vi "VMI_acquire_rewrite.vi"(0 "IO settings":T1, 1 "Queue Array":T7[](array[typedef]), 3 "Peak Find Settings":T5, 9 "Collection Information":T6[](array[typedef]), 11 "error in":errorcluster, 12 "Collect_refs":T4, 14 "Big_image Array":i16[][][](array[numeric])) -> (4 "Histogram":i32[][](array[numeric]), 6 "Peak Array":cluster{"X":sgl, "Y":sgl}[][](array[cluster]), 8 "Powers":dbl[][](array[numeric]), 10 "Power Err":dbl[][](array[numeric]), 15 "error IO":errorcluster)   [LabVIEW 2015]
doc: "This VI collects the images, finds the number of counts in each image"
uses:
  Type defs/FileAcq_v1_Ctrl.ctl
  Type defs/VMI_collection_refs.ctl
  Type defs/IO_settings_ctrl.ctl
  <vilib>/vision/Image Controls.llb/IMAQ Image.ctl
  <vilib>/userdefined/High Color/IMAQdx.ctl
panel:
  out "xaxis":i32[][](array[numeric])
  out "XY Graph":cluster{"Y":dbl[], "Y":dbl[]}[](graph)
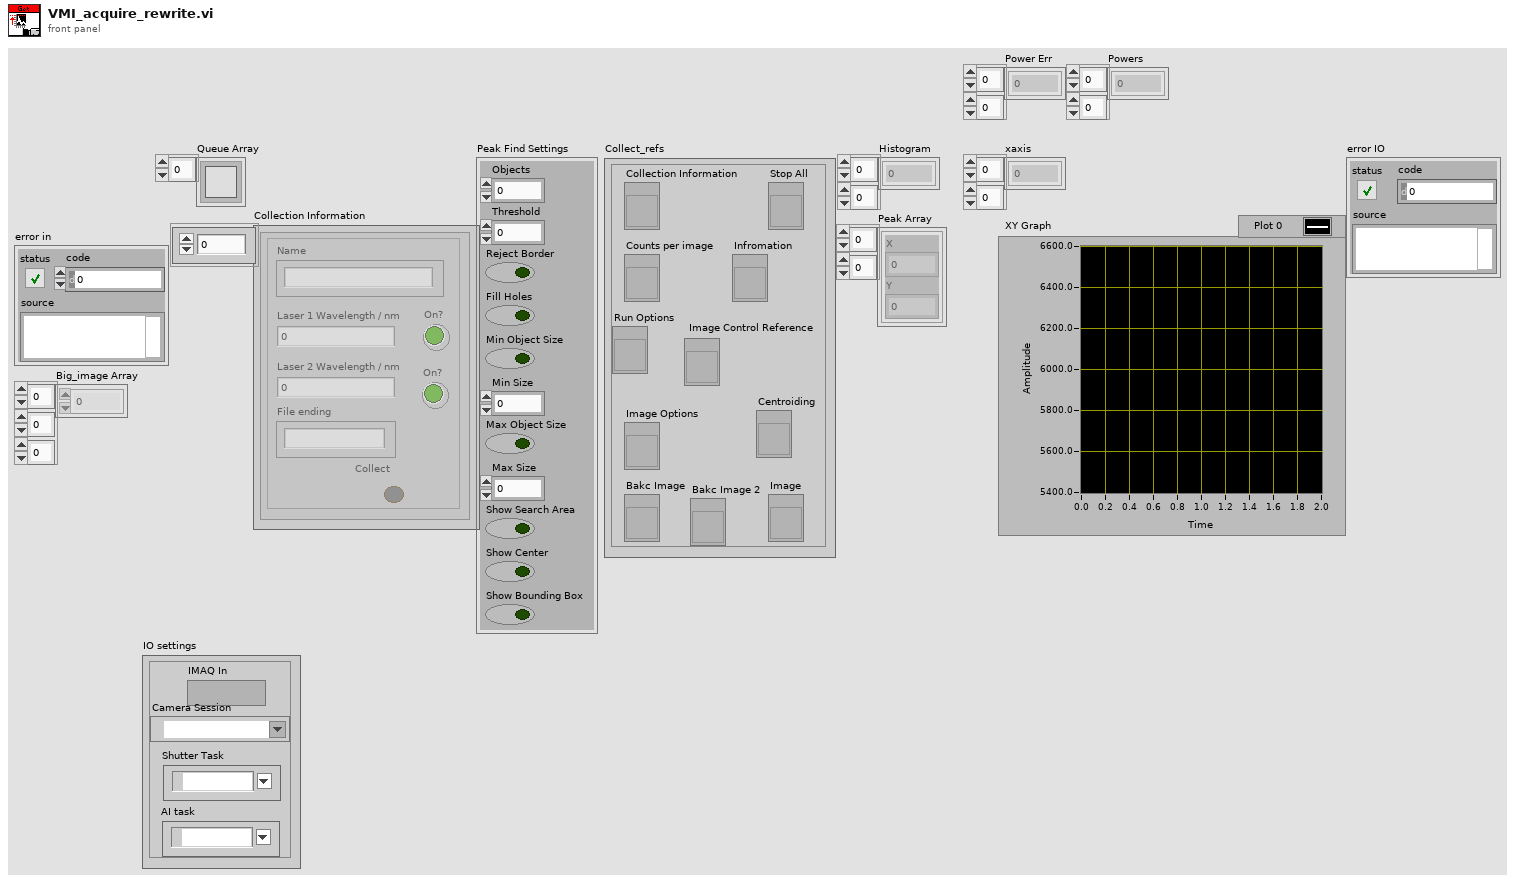
[diagram p1: front panel]
types:
  T1 = typedef "IO_settings_ctrl.ctl" = cluster{"IMAQ In":T2, "Camera Session":T3, "Shutter Task":refnum<k21>, "AI task":refnum<k21>}
  T2 = typedef "IMAQ Image.ctl" = refnum<image>
  T3 = typedef "IMAQdx.ctl" = refnum<k21>
  T4 = typedef "VMI_collection_refs.ctl" = cluster{"Stop All":refnum<vi>, "Collection Information ":refnum<vi>, "Infromation":refnum<vi>, "Counts per image":refnum<vi>, " Image Control Reference ":refnum<vi>, "Run Options":refnum<vi>, "Image Options":refnum<vi>, "Centroiding":refnum<vi>, "Image":refnum<vi>, "Bakc Image":refnum<vi>, "Bakc Image 2":refnum<vi>}
  T5 = cluster{"Objects":u16, "Threshold":i32, "Reject Border":bool, "Fill Holes":bool, "Min Object Size":bool, "Min Size":i32, "Max Object Size":bool, "Max Size":i32, "Show Search Area":bool, "Show Center":bool, "Show Bounding Box":bool}
  T6 = typedef "FileAcq_v1_Ctrl.ctl" = cluster{"Type":string, "LaserWave1":dbl, "Shutter1":bool, "LaserWave2":dbl, "Shutter2":bool, "FileEnd":string, "Collect":bool}
  T7 = typedef "Queue RefNum" = refnum<k1>
  T8 = typedef "Image Type" = u32
  T9 = cluster{"Total Time / ms":dbl, "Image Total Collection Time":dbl, "Image Loop time / ms":dbl, "Peak Total Find Time":dbl, "Peak Find Time / ms":dbl, "Camera Rate / Hz":dbl, "Total Number of Loops":dbl, "Current Loop Number":dbl, "Number of Image Loops":dbl, "Run Mode":dbl}
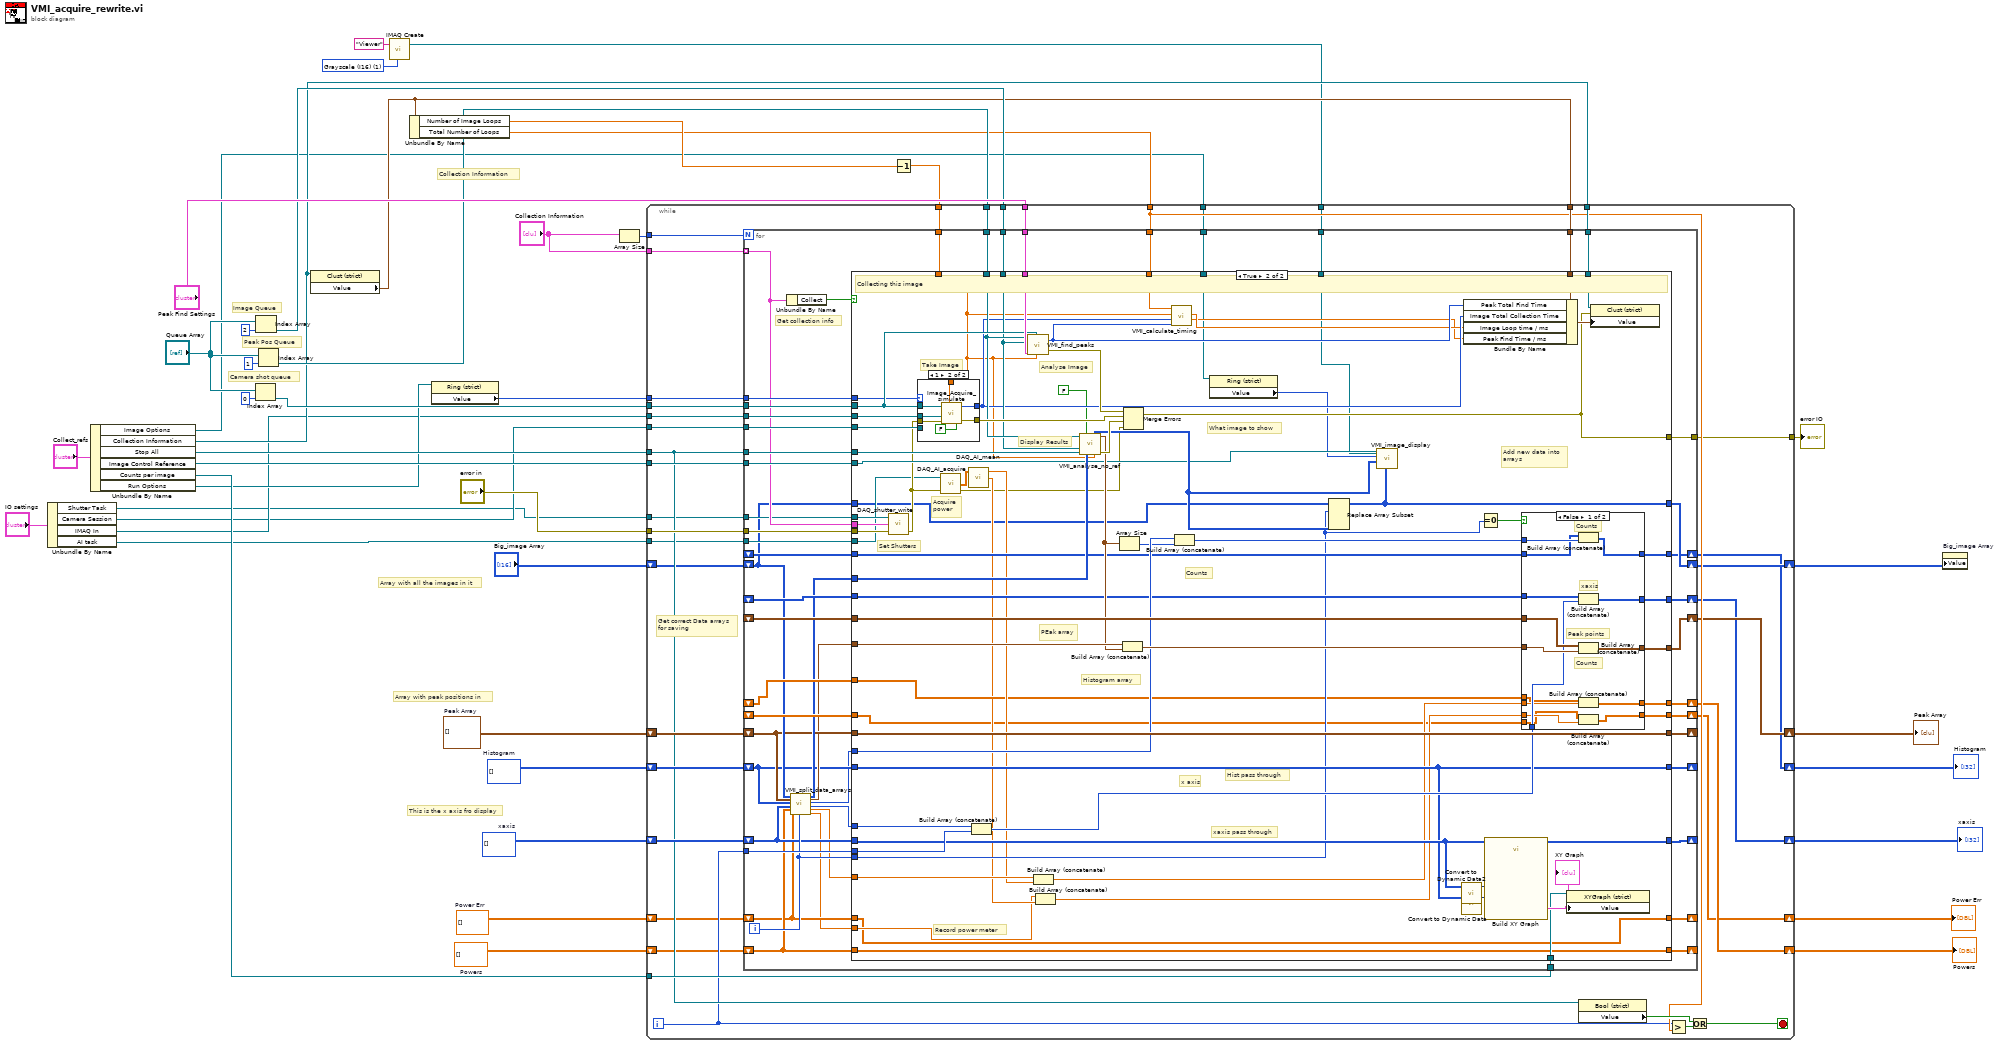
[diagram p0: block diagram]
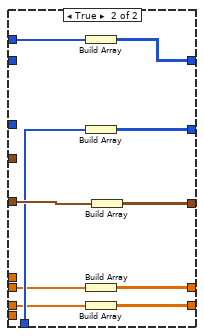
[diagram p3: hidden frame]
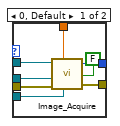
[diagram p4: hidden frame]
diagram:
  w3 = dbl[][] []  # Power Err
  w4 = dbl[][] []  # Powers
  w13 = T8 1 items=["Grayscale (U8)", "Grayscale (I16)", "Grayscale (SGL)", "Complex (CSG)", "RGB (U32)", "HSL (U32)", "RGB (U64)", "Grayscale (U16)"] ("Image Type")
  w5 = i32[][] []  # xaxis
  w23 = i32[][] []  # Histogram
  w25 = cluster{"X":sgl, "Y":sgl}[][] []  # Peak Array
  # "Array with all the images in it"
  # "Array with peak positions in"
  # "This is the x axis fro display"
  # "Collection Information"
  # "Image Queue"
  # "Peak Pos Queue"
  # "Camera shot queue"
  n1 = Unbundle By Name("IO settings") -> ("Shutter Task"=w7:refnum<k21>, "Camera Session"=w8:T3, "IMAQ In"=w9:T2, "AI task"=w6:refnum<k21>)
  n2 = Unbundle By Name("Collect_refs") -> ("Image Options"=w11:refnum<vi>, "Collection Information"=w27:refnum<vi>, "Stop All"=w33:refnum<vi>, "Image Control Reference"=w32:refnum<vi>, "Counts per image"=w24:refnum<vi>, "Run Options"=w16:refnum<vi>)
  n3 = Index Array(array="Queue Array", index=0) -> (element=w42:T7)
  n4 = Index Array(array="Queue Array", index=2) -> (element=w35:T7)
  n5 = Index Array(array="Queue Array", index=1) -> (element=w38:T7)
  n6 = property class="Clust (strict)"(reference=w27) -> ("Value"=w28:T9)  [unwired: 1 in, 2 out]
  n7 = call "IMAQ Create"("Image Name"="Viewer", "Image Type"=w13) -> ("New Image"=w12:T2)  [unwired: 3 in, 1 out]
  n8 = Unbundle By Name(w28) -> ("Number of Image Loops"=w31:dbl, "Total Number of Loops"=w29:dbl)
  n9 = property class="Ring (strict)"(reference=w16) -> ("Value"=w15:u16)  [unwired: 1 in, 2 out]
  n10 = Array Size(array="Collection Information") -> (size(s)=w26:i32)
  n11 = Decrement(x=w31) -> (x-1=w30:dbl)
  n12 = while {
    tunnel: w9 -> [w82]
    tunnel: w8 -> [w81]
    tunnel: "error in" -> [w80]
    tunnel: w42 -> [w79]
    tunnel: "Collection Information" -> [w78]
    tunnel: "Peak Find Settings" -> [w77]
    tunnel: w38 -> [w76]
    tunnel: w35 -> [w75]
    tunnel: w33 -> [w66]
    tunnel: w32 -> [w74]
    tunnel: w30 -> [w73]
    tunnel: w29 -> [w63]
    tunnel: w28 -> [w72]
    tunnel: w27 -> [w71]
    tunnel: w26 -> [w56]
    tunnel: w24 -> [w68]
    shift-right: [w55] -> w17
    shift-left: w25 -> [w70]
    shift-right: [w54] -> w18
    shift-left: w23 -> [w67]
    shift-right: [w53] -> w22
    shift-left: w5 -> [w69]
    tunnel: [w62] -> w21
    shift-right: [w61] -> w19
    shift-left: "Big_image Array" -> [w59]
    tunnel: w15 -> [w58]
    tunnel: w12 -> [w52]
    tunnel: w11 -> [w51]
    tunnel: w7 -> [w50]
    tunnel: w6 -> [w49]
    shift-right: [w46] -> w1
    shift-left: w4 -> [w48]
    shift-right: [w45] -> w2
    shift-left: w3 -> [w47]
    i -> [w60]
    stop <- w57 stop-if-true
    # "Get correct Data arrays\nfor saving"
    n13 = for {
      N: w56 -> [_]
      tunnel: w82 -> [w134]
      tunnel: w81 -> [w133]
      tunnel: w80 -> [w132]
      tunnel: w79 -> [w131]
      tunnel: w78 -> [w104] mode=indexing
      tunnel: w77 -> [w129]
      tunnel: w76 -> [w128]
      tunnel: w75 -> [w127]
      tunnel: w66 -> [w126]
      tunnel: w74 -> [w125]
      tunnel: w73 -> [w123]
      tunnel: w63 -> [w122]
      tunnel: w60 -> [w119]
      tunnel: w72 -> [w121]
      tunnel: w71 -> [w120]
      tunnel: w68 -> [w118]
      shift-right: [w117] -> _
      shift-left: w70 -> [w92]
      shift-right: [w124] -> _
      shift-left: w67 -> [w90]
      shift-right: [w116] -> _
      shift-left: w69 -> [w88]
      tunnel: [w115] -> w62
      shift-right: [w114] -> w61
      shift-left: w59 -> [w94]
      tunnel: w58 -> [w113]
      shift-right: [w112] -> w55
      shift-left: _ -> [w111]
      shift-right: [w110] -> w54
      shift-left: _ -> [w109]
      shift-right: [w108] -> w53
      shift-left: _ -> [w107]
      tunnel: w52 -> [w106]
      tunnel: w51 -> [w105]
      tunnel: w50 -> [w103]
      tunnel: w49 -> [w102]
      shift-right: [w101] -> _
      shift-left: w48 -> [w86]
      shift-right: [w100] -> w46
      shift-left: _ -> [w99]
      shift-right: [w98] -> _
      shift-left: w47 -> [w85]
      shift-right: [w97] -> w45
      shift-left: _ -> [w96]
      i -> [w95]
      # "Get collection info"
      # "This loop collects for each required image"
      n14 = Unbundle By Name(w104) -> ("Collect"=w130:bool)
      n15 = call "VMI_split_data_arrays.vi"("Big_image Array in"=w94, "Peak Array in"=w92, "Histogram in"=w90, "xaxis in"=w88, "Powers in"=w86, "Power Err in"=w85, "ArrayIndex"=w95) -> ("Big_image Array out"=w93:i16[][], "Peak Array out"=w91:cluster{"X":sgl, "Y":sgl}[], "Histogram out"=w89:i32[], "xaxis out"=w87:i32[], "Powers out"=w84:dbl[], "Power Err out"=w83:dbl[])  [unwired: 7 in]
      n16 = case shown="True" w130 {
        tunnel: w134 -> [_ w216]
        tunnel: w133 -> [_ w215]
        tunnel: w132 -> [w143 w163]
        tunnel: w131 -> [_ w213]
        tunnel: w129 -> [_ w214]
        tunnel: w128 -> [_ w210]
        tunnel: w127 -> [_ w209]
        tunnel: w126 -> [_ w208]
        tunnel: w125 -> [_ w168]
        tunnel: [w143 w196] -> w115
        tunnel: w91 -> [_ w185]
        tunnel: w92 -> [w141 w186]
        tunnel: [w141 w186] -> w117
        tunnel: w90 -> [w140 w171]
        tunnel: w89 -> [_ w182]
        tunnel: [w140 w171] -> w124
        tunnel: w123 -> [_ w190]
        tunnel: w122 -> [_ w207]
        tunnel: w119 -> [_ w173]
        tunnel: w87 -> [_ w175]
        tunnel: w88 -> [w139 w172]
        tunnel: [w139 w172] -> w116
        tunnel: w121 -> [_ w203]
        tunnel: w120 -> [_ w197]
        tunnel: w95 -> [_ w169]
        tunnel: w118 -> [_ w194]
        tunnel: w94 -> [w142 w145]
        tunnel: [w142 w144] -> w114
        tunnel: w93 -> [_ w193]
        tunnel: w113 -> [_ w192]
        tunnel: [w141 w188] -> w112
        tunnel: w111 -> [_ w187]
        tunnel: [w140 w179] -> w110
        tunnel: w109 -> [_ w178]
        tunnel: [w139 w177] -> w108
        tunnel: w107 -> [_ w176]
        tunnel: w106 -> [_ w167]
        tunnel: w105 -> [_ w166]
        tunnel: w104 -> [_ w164]
        tunnel: w103 -> [_ w162]
        tunnel: w102 -> [_ w160]
        tunnel: w84 -> [_ w157]
        tunnel: w86 -> [w138 w158]
        tunnel: [w138 w158] -> w101
        tunnel: [w136 w155] -> w100
        tunnel: w99 -> [w136 w154]
        tunnel: w83 -> [_ w151]
        tunnel: w85 -> [w137 w150]
        tunnel: [w137 w150] -> w98
        tunnel: [w135 w148] -> w97
        tunnel: w96 -> [w135 w147]
        frame False {
          # "Not collecting this image"
        }
        frame True {
          # "xaxis pass through"
          # "Hist pass through"
          # "Acquire\npower"
          # "Record power meter"
          # "Set Shutters"
          # "What image to show"
          # "x axis"
          # "Histogram array"
          # "PEak array"
          # "Counts"
          # "Add new data into\narrays"
          # "Display Results"
          # "Analyse Image"
          # "Take Image"
          # "Collecting this image"
          n17 = call "DAQ_shutter_write.vi"("Error In"=w163, "Collection Settings"=w164, "DAQmx Task Name"=w162) -> ("Error Out"=w161:errorcluster)  [unwired: 2 in]
          n18 = case shown="1" w192 {
            tunnel: w216 -> [w248 w250]
            tunnel: w215 -> [w247 _]
            tunnel: w161 -> [w246 w256]
            tunnel: w213 -> [w245 w252]
            tunnel: [w244 w255] -> w211
            tunnel: w190 -> [w243 w253]
            tunnel: [w242 w254] -> w201
            frame 0, Default {
              n19 = call "Image_Acquire.vi"("Queue Ref in"=w245, "Acquire Time"=w243, "Image Out"=w248, "Session In"=w247, "error in (no error)"=w246, "Test Timing"=FALSE) -> ("Loop Time Out"=w242:i64, "error out"=w244:errorcluster)  [unwired: 1 in]
            }
            frame 1 {
              n20 = call "Image_Acquire_simulate.vi"("Queue Ref in"=w252, "Acquire Time"=w253, "Image Out"=w250, "error in (no error)"=w256, "Test Timing"=FALSE) -> ("Loop Time Out"=w254:i64, "error out"=w255:errorcluster)  [unwired: 2 in]
            }
          }
          n21 = call "DAQ_AI_acquire.vi"("Error In"=w161, "DAQmx Task Name"=w160) -> ("Error Out"=w146:errorcluster, "data"=w159:dbl[][])  [unwired: 1 in, 1 out]
          n22 = call "DAQ_AI_mean.vi"("data"=w159) -> ("Std"=w152:dbl[], "Mean"=w156:dbl[])  [unwired: 3 in]
          n23 = Build Array (concatenate)(w175, w173) -> (w174:i32[])
          n24 = call "VMI_find_peaks.vi"("Acquire Time"=w190, "Acquire Queue In"=w213, "Peak Find Settings"=w214, "Image Queue in"=w209, "Peak Position Queue in"=w210) -> ("error out"=w212:errorcluster, "x-y"=w202:u32)  [unwired: 1 in]
          n25 = Build Array (concatenate)(w157, w156) -> (w153:dbl[])
          n26 = Build Array (concatenate)(w151, w152) -> (w149:dbl[])
          n27 = call "VMI_analyse_no_ref.vi"("Peak Position Queue in"=w210, "Test Timing"=FALSE, "Image in"=w209, "Stop Button Ref"=w208, "Image_array"=w193, "Acquire Time"=w190) -> ("Image_array out"=w170:i32[][], "Peaks Position Out"=w184:cluster{"X":sgl, "Y":sgl}[], "error out"=w205:errorcluster)  [unwired: 5 in, 2 out]
          n28 = Array Size(array=w184) -> (size(s)=w181:i32)
          n29 = Build Array (concatenate)(w185, w184) -> (w183:cluster{"X":sgl, "Y":sgl}[])
          n30 = Merge Errors(w212, w211, w205, w146) -> (w196:errorcluster)
          n31 = call "VMI_calculate_timing.vi"("Peakfind total time"=w202, "Camera_Total_loop time"=w201, "Number of image loops"=w190, "Total loop Number"=w207) -> ("AveragePeak find time"=w199:dbl, "Average Image Loop time"=w200:dbl)  [unwired: 1 in, 1 out]
          n32 = Build Array (concatenate)(w182, w181) -> (w180:i32[])
          n33 = property class="Ring (strict)"(reference=w166) -> ("Value"=w165:u16)  [unwired: 1 in, 2 out]
          n34 = Replace Array Subset(array=w145, new element=w170, index (dim 0)=w169) -> (w144:i16[][][])  [unwired: 2 in]
          n35 = call "VMI_image_display.vi"("Image_control"=w168, "Image to show"=w165, "Current Image"=w170, "Big_image Array"=w144, "Canvas"=w167) -> ()  [unwired: 5 in, 1 out]
          n36 = call "Convert to Dynamic Data2"("2D Array"=w172) -> ("Dynamic Data Type"=w204:dynamicdata)  [unwired: 3 in]
          n37 = call "Convert to Dynamic Data"("2D Array"=w171) -> ("Dynamic Data Type"=w206:dynamicdata)  [unwired: 3 in]
          n38 = Bundle By Name(cluster=w203, "Peak Total Find Time"=w202, "Image Total Collection Time"=w201, "Image Loop time / ms"=w200, "Peak Find Time / ms"=w199) -> (w198:T9)
          n39 = Equal To 0?(x=w169) -> (x = 0?=w189:bool)
          n40 = call "Build XY Graph"("Y Input"=w206, "X Input"=w204) -> ("XY Graph"=w195:cluster{"X":dbl[], "Y":dbl[]}[])  [unwired: 8 in, 1 out]
          "XY Graph" <- w195
          n41 = case shown="False" w189 {
            tunnel: w183 -> [w231 w241]
            tunnel: [w230 w240] -> w188
            tunnel: w187 -> [w229 _]
            tunnel: w180 -> [w228 w239]
            tunnel: [w227 w238] -> w179
            tunnel: w178 -> [w226 _]
            tunnel: w174 -> [w225 w236]
            tunnel: [w224 w237] -> w177
            tunnel: w176 -> [w223 _]
            tunnel: w153 -> [w221 w235]
            tunnel: [w220 w234] -> w155
            tunnel: w154 -> [w222 _]
            tunnel: w149 -> [w219 w233]
            tunnel: [w218 w232] -> w148
            tunnel: w147 -> [w217 _]
            frame False {
              # "Counts"
              # "Counts"
              # "Peak points"
              # "xaxis"
              n42 = Build Array (concatenate)(w226, w228) -> (w227:i32[][])
              n43 = Build Array (concatenate)(w223, w225) -> (w224:i32[][])
              n44 = Build Array (concatenate)(w229, w231) -> (w230:cluster{"X":sgl, "Y":sgl}[][])
              n45 = Build Array (concatenate)(w222, w221) -> (w220:dbl[][])
              n46 = Build Array (concatenate)(w217, w219) -> (w218:dbl[][])
            }
            frame True {
              n47 = Build Array(w239) -> (w238:i32[][])
              n48 = Build Array(w236) -> (w237:i32[][])
              n49 = Build Array(w235) -> (w234:dbl[][])
              n50 = Build Array(w233) -> (w232:dbl[][])
              n51 = Build Array(w241) -> (w240:cluster{"X":sgl, "Y":sgl}[][])
            }
          }
          n52 = property on="Property Node" class="XYGraph (strict)"(reference=w194, "Value"=w195) -> ()  [unwired: 1 in, 2 out]
          n53 = property class="Clust (strict)"(reference=w197, error in=w196, "Value"=w198) -> ()  [unwired: 2 out]
        }
      }
    }
    n54 = property on="Property Node" class="Bool (strict)"(reference=w66) -> ("Value"=w65:bool)  [unwired: 1 in, 2 out]
    n55 = Greater?(x=w60, y=w63) -> (0:w64:bool)
    n56 = Or(x=w65, y=w64) -> (x .or. y?=w57:bool)
  }
  "Histogram" <- w18
  "Peak Array" <- w17
  "xaxis" <- w22
  "error IO" <- w21
  "Power Err" <- w2
  "Powers" <- w1
  n57 = property on="Big_image Array" class="Arr (strict)"("Value"=w19) -> ()  [unwired: 2 in, 2 out]
